vi "GradeProtocol.vi"() -> (1 "GradeProtocol":string, 2 "output 1":i32, 3 "outputProtocol":string)   [LabVIEW 2018]
uses:
  Global Variables.vi
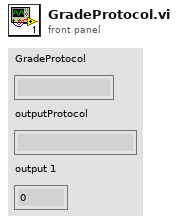
[diagram p1: front panel]
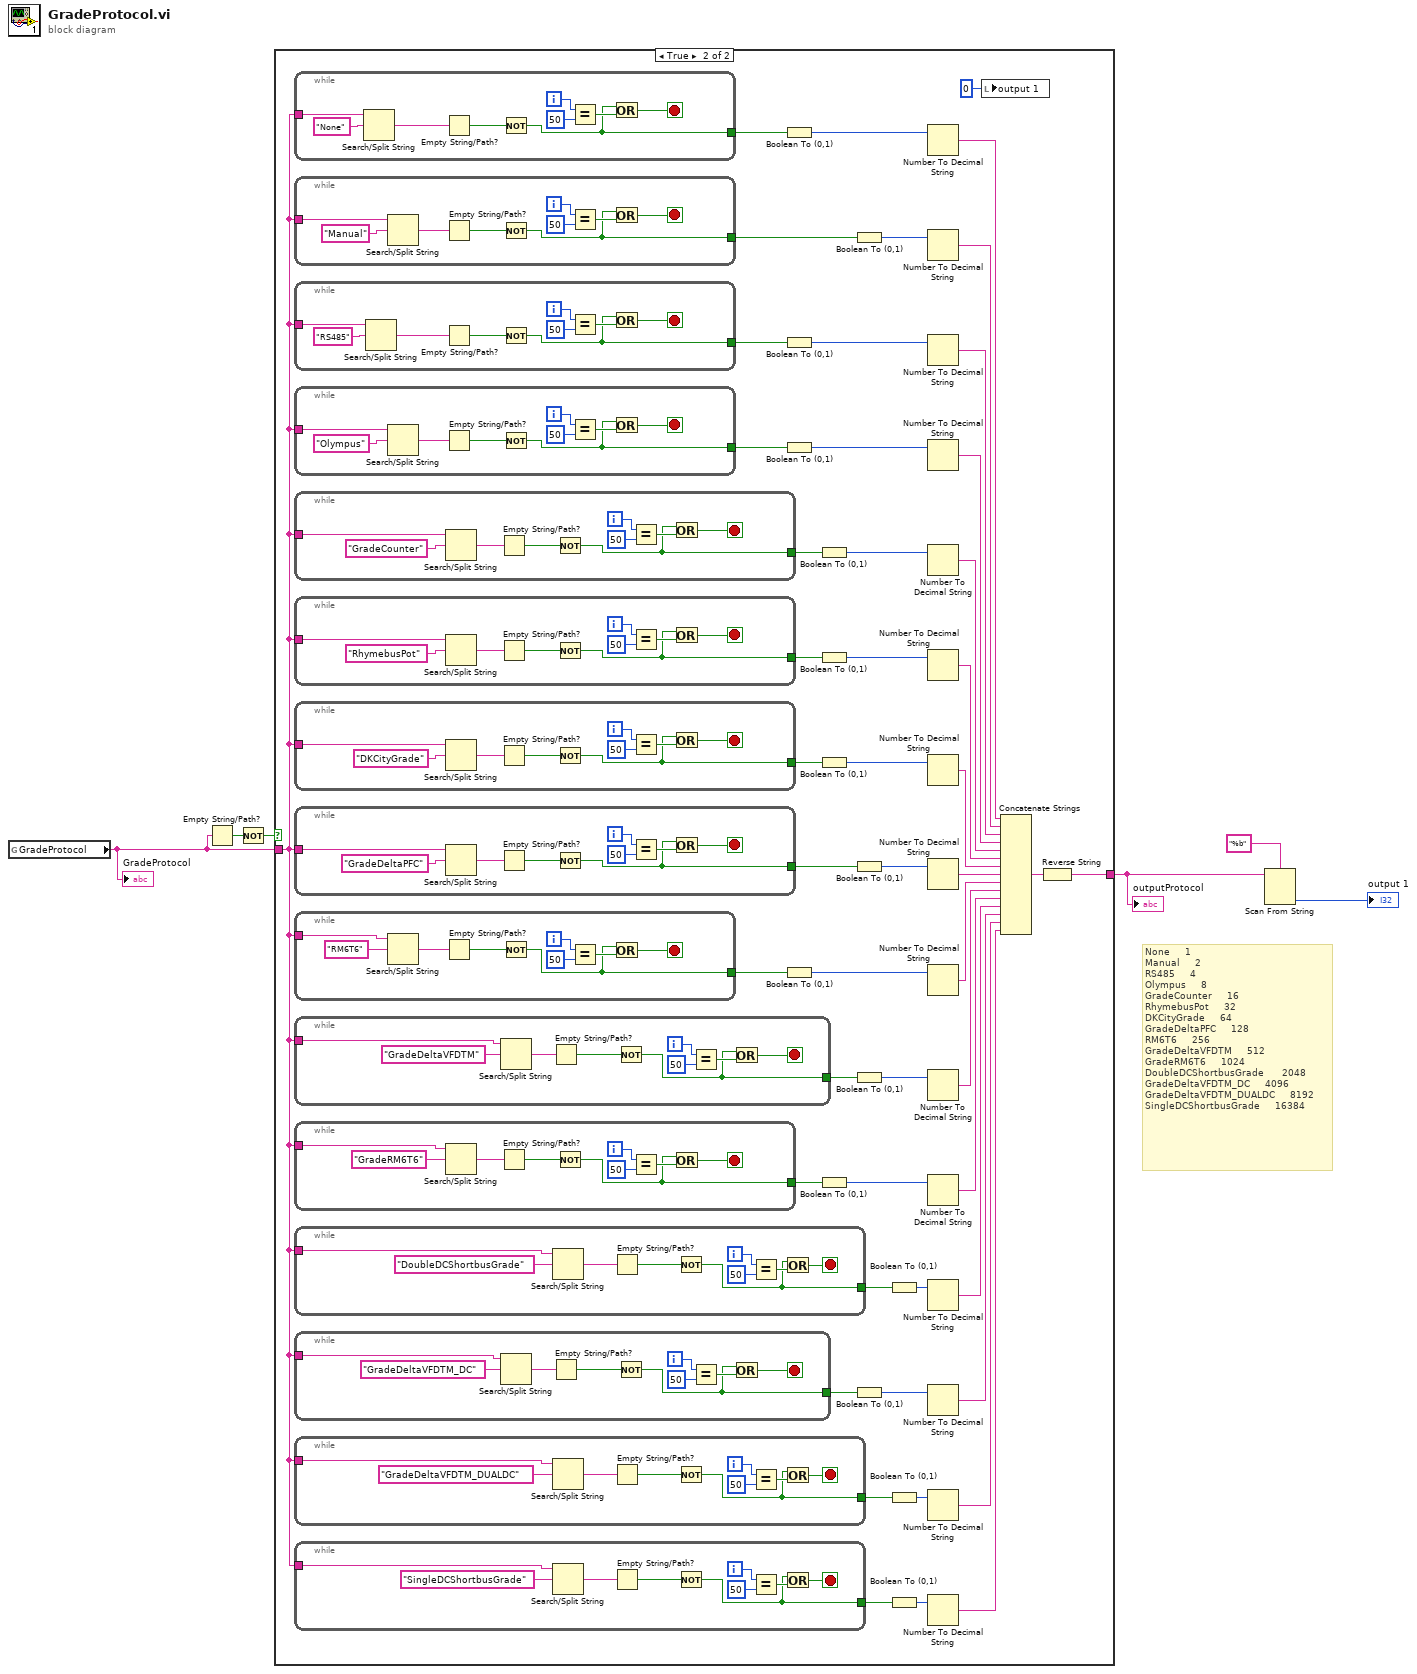
[diagram p0: block diagram]
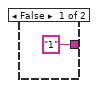
[diagram p2: hidden frame]
diagram:
  # "None     1\nManual     2\nRS485     4\nOlympus     8\nGradeCounter     16\nRhymebusPot     32\nDKCityGrade     64\nGradeDeltaPFC     128\nRM6T6     256\nGradeDeltaVFDTM     512\nGradeRM6T6     1024\nDoubleDCShortbusGrade      2048\nGradeDeltaVFDTM_DC     4096\nGradeDeltaVFDTM_DUALDC     8192\nSingleDCShortbusGrade     16384"
  n1 = global read "Global Variables.vi" "GradeProtocol"() -> (w2:string)
  "GradeProtocol" <- w2
  n2 = Empty String/Path?(string/path=w2) -> (empty?=w3:bool)
  n3 = Not(x=w3) -> (.not. x?=w1:bool)
  n4 = case shown="True" w1 {
    tunnel: w2 -> [_ w28]
    tunnel: ["1" w9] -> w5
    frame False {
    }
    frame True {
      n5 = while {
        tunnel: w28 -> [w187]
        tunnel: [w183] -> w55
        i -> [w191]
        stop <- w189 stop-if-true
        n6 = Search/Split String(string=w187, search string/char (-)="None") -> (match + rest of string=w184:string)  [unwired: 1 in, 2 out]
        n7 = Empty String/Path?(string/path=w184) -> (empty?=w185:bool)
        n8 = Not(x=w185) -> (.not. x?=w183:bool)
        n9 = Equal?(x=w191, y=50) -> (x = y?=w188:bool)
        n10 = Or(x=w183, y=w188) -> (x .or. y?=w189:bool)
      }
      n11 = while {
        tunnel: w28 -> [w178]
        tunnel: [w174] -> w46
        i -> [w182]
        stop <- w180 stop-if-true
        n12 = Search/Split String(string=w178, search string/char (-)="Manual") -> (match + rest of string=w175:string)  [unwired: 1 in, 2 out]
        n13 = Empty String/Path?(string/path=w175) -> (empty?=w176:bool)
        n14 = Not(x=w176) -> (.not. x?=w174:bool)
        n15 = Equal?(x=w182, y=50) -> (x = y?=w179:bool)
        n16 = Or(x=w174, y=w179) -> (x .or. y?=w180:bool)
      }
      n17 = while {
        tunnel: w28 -> [w169]
        tunnel: [w165] -> w45
        i -> [w173]
        stop <- w171 stop-if-true
        n18 = Search/Split String(string=w169, search string/char (-)="RS485") -> (match + rest of string=w166:string)  [unwired: 1 in, 2 out]
        n19 = Empty String/Path?(string/path=w166) -> (empty?=w167:bool)
        n20 = Not(x=w167) -> (.not. x?=w165:bool)
        n21 = Equal?(x=w173, y=50) -> (x = y?=w170:bool)
        n22 = Or(x=w165, y=w170) -> (x .or. y?=w171:bool)
      }
      n23 = while {
        tunnel: w28 -> [w160]
        tunnel: [w156] -> w44
        i -> [w164]
        stop <- w162 stop-if-true
        n24 = Search/Split String(string=w160, search string/char (-)="Olympus") -> (match + rest of string=w157:string)  [unwired: 1 in, 2 out]
        n25 = Empty String/Path?(string/path=w157) -> (empty?=w158:bool)
        n26 = Not(x=w158) -> (.not. x?=w156:bool)
        n27 = Equal?(x=w164, y=50) -> (x = y?=w161:bool)
        n28 = Or(x=w156, y=w161) -> (x .or. y?=w162:bool)
      }
      n29 = while {
        tunnel: w28 -> [w151]
        tunnel: [w147] -> w43
        i -> [w155]
        stop <- w153 stop-if-true
        n30 = Search/Split String(string=w151, search string/char (-)="GradeCounter") -> (match + rest of string=w148:string)  [unwired: 1 in, 2 out]
        n31 = Empty String/Path?(string/path=w148) -> (empty?=w149:bool)
        n32 = Not(x=w149) -> (.not. x?=w147:bool)
        n33 = Equal?(x=w155, y=50) -> (x = y?=w152:bool)
        n34 = Or(x=w147, y=w152) -> (x .or. y?=w153:bool)
      }
      n35 = while {
        tunnel: w28 -> [w142]
        tunnel: [w138] -> w42
        i -> [w146]
        stop <- w144 stop-if-true
        n36 = Search/Split String(string=w142, search string/char (-)="RhymebusPot") -> (match + rest of string=w139:string)  [unwired: 1 in, 2 out]
        n37 = Empty String/Path?(string/path=w139) -> (empty?=w140:bool)
        n38 = Not(x=w140) -> (.not. x?=w138:bool)
        n39 = Equal?(x=w146, y=50) -> (x = y?=w143:bool)
        n40 = Or(x=w138, y=w143) -> (x .or. y?=w144:bool)
      }
      n41 = while {
        tunnel: w28 -> [w133]
        tunnel: [w129] -> w41
        i -> [w137]
        stop <- w135 stop-if-true
        n42 = Search/Split String(string=w133, search string/char (-)="DKCityGrade") -> (match + rest of string=w130:string)  [unwired: 1 in, 2 out]
        n43 = Empty String/Path?(string/path=w130) -> (empty?=w131:bool)
        n44 = Not(x=w131) -> (.not. x?=w129:bool)
        n45 = Equal?(x=w137, y=50) -> (x = y?=w134:bool)
        n46 = Or(x=w129, y=w134) -> (x .or. y?=w135:bool)
      }
      n47 = while {
        tunnel: w28 -> [w124]
        tunnel: [w120] -> w40
        i -> [w128]
        stop <- w126 stop-if-true
        n48 = Search/Split String(string=w124, search string/char (-)="GradeDeltaPFC") -> (match + rest of string=w121:string)  [unwired: 1 in, 2 out]
        n49 = Empty String/Path?(string/path=w121) -> (empty?=w122:bool)
        n50 = Not(x=w122) -> (.not. x?=w120:bool)
        n51 = Equal?(x=w128, y=50) -> (x = y?=w125:bool)
        n52 = Or(x=w120, y=w125) -> (x .or. y?=w126:bool)
      }
      n53 = while {
        tunnel: w28 -> [w115]
        tunnel: [w111] -> w39
        i -> [w119]
        stop <- w117 stop-if-true
        n54 = Search/Split String(string=w115, search string/char (-)="RM6T6") -> (match + rest of string=w112:string)  [unwired: 1 in, 2 out]
        n55 = Empty String/Path?(string/path=w112) -> (empty?=w113:bool)
        n56 = Not(x=w113) -> (.not. x?=w111:bool)
        n57 = Equal?(x=w119, y=50) -> (x = y?=w116:bool)
        n58 = Or(x=w111, y=w116) -> (x .or. y?=w117:bool)
      }
      n59 = while {
        tunnel: w28 -> [w106]
        tunnel: [w102] -> w21
        i -> [w110]
        stop <- w108 stop-if-true
        n60 = Search/Split String(string=w106, search string/char (-)="GradeDeltaVFDTM") -> (match + rest of string=w103:string)  [unwired: 1 in, 2 out]
        n61 = Empty String/Path?(string/path=w103) -> (empty?=w104:bool)
        n62 = Not(x=w104) -> (.not. x?=w102:bool)
        n63 = Equal?(x=w110, y=50) -> (x = y?=w107:bool)
        n64 = Or(x=w102, y=w107) -> (x .or. y?=w108:bool)
      }
      n65 = while {
        tunnel: w28 -> [w97]
        tunnel: [w93] -> w20
        i -> [w101]
        stop <- w99 stop-if-true
        n66 = Search/Split String(string=w97, search string/char (-)="GradeRM6T6") -> (match + rest of string=w94:string)  [unwired: 1 in, 2 out]
        n67 = Empty String/Path?(string/path=w94) -> (empty?=w95:bool)
        n68 = Not(x=w95) -> (.not. x?=w93:bool)
        n69 = Equal?(x=w101, y=50) -> (x = y?=w98:bool)
        n70 = Or(x=w93, y=w98) -> (x .or. y?=w99:bool)
      }
      n71 = while {
        tunnel: w28 -> [w88]
        tunnel: [w84] -> w19
        i -> [w92]
        stop <- w90 stop-if-true
        n72 = Search/Split String(string=w88, search string/char (-)="DoubleDCShortbusGrade") -> (match + rest of string=w85:string)  [unwired: 1 in, 2 out]
        n73 = Empty String/Path?(string/path=w85) -> (empty?=w86:bool)
        n74 = Not(x=w86) -> (.not. x?=w84:bool)
        n75 = Equal?(x=w92, y=50) -> (x = y?=w89:bool)
        n76 = Or(x=w84, y=w89) -> (x .or. y?=w90:bool)
      }
      n77 = while {
        tunnel: w28 -> [w79]
        tunnel: [w75] -> w18
        i -> [w83]
        stop <- w81 stop-if-true
        n78 = Search/Split String(string=w79, search string/char (-)="GradeDeltaVFDTM_DC") -> (match + rest of string=w76:string)  [unwired: 1 in, 2 out]
        n79 = Empty String/Path?(string/path=w76) -> (empty?=w77:bool)
        n80 = Not(x=w77) -> (.not. x?=w75:bool)
        n81 = Equal?(x=w83, y=50) -> (x = y?=w80:bool)
        n82 = Or(x=w75, y=w80) -> (x .or. y?=w81:bool)
      }
      n83 = while {
        tunnel: w28 -> [w61]
        tunnel: [w57] -> w17
        i -> [w65]
        stop <- w63 stop-if-true
        n84 = Search/Split String(string=w61, search string/char (-)="GradeDeltaVFDTM_DUALDC") -> (match + rest of string=w58:string)  [unwired: 1 in, 2 out]
        n85 = Empty String/Path?(string/path=w58) -> (empty?=w59:bool)
        n86 = Not(x=w59) -> (.not. x?=w57:bool)
        n87 = Equal?(x=w65, y=50) -> (x = y?=w62:bool)
        n88 = Or(x=w57, y=w62) -> (x .or. y?=w63:bool)
      }
      n89 = while {
        tunnel: w28 -> [w70]
        tunnel: [w66] -> w16
        i -> [w74]
        stop <- w72 stop-if-true
        n90 = Search/Split String(string=w70, search string/char (-)="SingleDCShortbusGrade") -> (match + rest of string=w67:string)  [unwired: 1 in, 2 out]
        n91 = Empty String/Path?(string/path=w67) -> (empty?=w68:bool)
        n92 = Not(x=w68) -> (.not. x?=w66:bool)
        n93 = Equal?(x=w74, y=50) -> (x = y?=w71:bool)
        n94 = Or(x=w66, y=w71) -> (x .or. y?=w72:bool)
      }
      n95 = Boolean To (0,1)(Boolean=w55) -> (0, 1=w56:i16)
      n96 = Boolean To (0,1)(Boolean=w45) -> (0, 1=w53:i16)
      n97 = Boolean To (0,1)(Boolean=w44) -> (0, 1=w52:i16)
      n98 = Boolean To (0,1)(Boolean=w39) -> (0, 1=w48:i16)
      n99 = Boolean To (0,1)(Boolean=w43) -> (0, 1=w51:i16)
      n100 = Boolean To (0,1)(Boolean=w42) -> (0, 1=w50:i16)
      n101 = Boolean To (0,1)(Boolean=w41) -> (0, 1=w49:i16)
      n102 = Boolean To (0,1)(Boolean=w20) -> (0, 1=w26:i16)
      n103 = Boolean To (0,1)(Boolean=w46) -> (0, 1=w54:i16)
      n104 = Boolean To (0,1)(Boolean=w40) -> (0, 1=w47:i16)
      n105 = Boolean To (0,1)(Boolean=w21) -> (0, 1=w27:i16)
      n106 = Boolean To (0,1)(Boolean=w18) -> (0, 1=w24:i16)
      n107 = Boolean To (0,1)(Boolean=w19) -> (0, 1=w25:i16)
      n108 = Boolean To (0,1)(Boolean=w17) -> (0, 1=w23:i16)
      n109 = Boolean To (0,1)(Boolean=w16) -> (0, 1=w22:i16)
      n110 = Number To Decimal String(number=w56) -> (decimal integer string=w38:string)  [unwired: 1 in]
      n111 = Number To Decimal String(number=w54) -> (decimal integer string=w37:string)  [unwired: 1 in]
      n112 = Number To Decimal String(number=w53) -> (decimal integer string=w36:string)  [unwired: 1 in]
      n113 = Number To Decimal String(number=w52) -> (decimal integer string=w35:string)  [unwired: 1 in]
      n114 = Number To Decimal String(number=w51) -> (decimal integer string=w34:string)  [unwired: 1 in]
      n115 = Number To Decimal String(number=w50) -> (decimal integer string=w33:string)  [unwired: 1 in]
      n116 = Number To Decimal String(number=w49) -> (decimal integer string=w32:string)  [unwired: 1 in]
      n117 = Number To Decimal String(number=w47) -> (decimal integer string=w31:string)  [unwired: 1 in]
      n118 = Number To Decimal String(number=w48) -> (decimal integer string=w30:string)  [unwired: 1 in]
      n119 = Number To Decimal String(number=w27) -> (decimal integer string=w15:string)  [unwired: 1 in]
      n120 = Number To Decimal String(number=w26) -> (decimal integer string=w14:string)  [unwired: 1 in]
      n121 = Number To Decimal String(number=w25) -> (decimal integer string=w13:string)  [unwired: 1 in]
      n122 = Number To Decimal String(number=w24) -> (decimal integer string=w12:string)  [unwired: 1 in]
      n123 = Number To Decimal String(number=w23) -> (decimal integer string=w11:string)  [unwired: 1 in]
      n124 = Number To Decimal String(number=w22) -> (decimal integer string=w10:string)  [unwired: 1 in]
      n125 = local write "output 1"(0 ("output 1")) -> ()
      n126 = Concatenate Strings(w38, w37, w36, w35, w34, w33, w32, w31, w30, w15, w14, w13, w12, w11, w10) -> (w29:string)
      n127 = Reverse String(1:w29) -> (0:w9:string)
    }
  }
  "outputProtocol" <- w5
  n128 = Scan From String(format string="%b", input string=w5) -> (output 1=→"output 1":i32)  [unwired: 3 in, 3 out]
